vi "Delete RT FIFO.vi"(8 "error in (no error)":errorcluster, 11 "rt fifo":refnum<k33>) -> (0 "error out":errorcluster)   [LabVIEW 2020, in "DSF Core.lvlib" / "Interface.lvclass"]
uses:
  Interface.lvclass
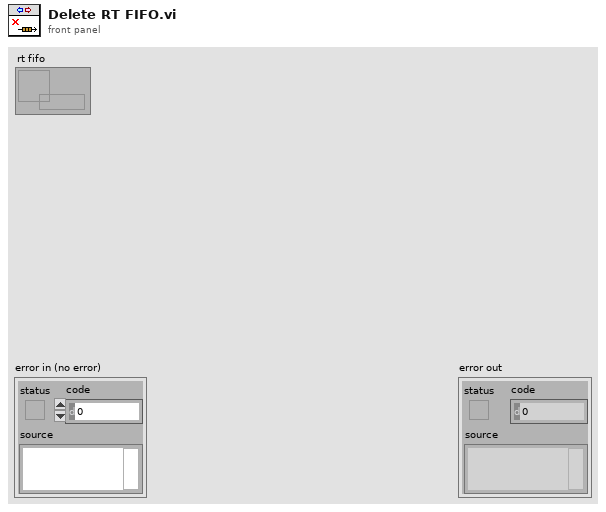
[diagram p1: front panel]
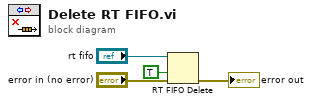
[diagram p0: block diagram]
diagram:
  n1 = RT FIFO Delete(0:"rt fifo", 2:TRUE ("force destroy? (F)"), 3:"error in (no error)") -> (11:→"error out":errorcluster)
